vi "PC-PLC.vi"() -> ()   [LabVIEW 2022 SP3]
uses:
  Labview/Globali.vi
panel:
  out "DB20.DBW 254":u16
  out "DB20.DBW 252":u16
  out "DB20.DBW 250":u16
  out "DB20.DBW 248":u16
  out "DB20.DBW 246":u16
  out "DB20.DBW 244":u16
  out "DB20.DBW 242":u16
  out "DB20.DBW 240":u16
  out "DB20.DBW 238":u16
  out "DB20.DBW 236":u16
  out "DB20.DBW 234":u16
  out "DB20.DBW 232":u16
  out "DB20.DBW 230":u16
  out "DB20.DBW 228":u16
  out "DB20.DBW 226":u16
  out "DB20.DBW 224":u16
  out "DB20.DBW 222":u16
  out "DB20.DBW 220":u16
  out "DB20.DBW 218":u16
  out "DB20.DBW 216":u16
  out "DB20.DBW 214":u16
  out "DB20.DBW 212":u16
  out "DB20.DBW 210":u16
  out "DB20.DBW 208":u16
  out "DB20.DBW 206":u16
  out "DB20.DBW 204":u16
  out "DB20.DBW 202":u16
  out "DB20.DBW 200":u16
  out "DB20.DBW 198":u16
  out "DB20.DBW 196":u16
  out "DB20.DBW 194":u16
  out "DB20.DBW 192":u16
  out "DB20.DBW 190":u16
  out "DB20.DBW 188":u16
  out "DB20.DBW 186":u16
  out "DB20.DBW 184":u16
  out "DB20.DBW 182":u16
  out "DB20.DBW 180":u16
  out "DB20.DBW 178":u16
  out "DB20.DBW 176":u16
  out "DB20.DBW 174":u16
  out "DB20.DBW 172":u16
  out "DB20.DBW 170":u16
  out "DB20.DBW 168":u16
  out "DB20.DBW 166":u16
  out "DB20.DBW 164":u16
  out "DB20.DBW 162":u16
  out "DB20.DBW 160":u16
  out "DB20.DBW 158":u16
  out "DB20.DBW 156":u16
  out "DB20.DBW 154":u16
  out "DB20.DBW 152":u16
  out "DB20.DBW 150":u16
  out "DB20.DBW 148":u16
  out "DB20.DBW 146":u16
  out "DB20.DBW 144":u16
  out "DB20.DBW 142":u16
  out "DB20.DBW 140":u16
  out "DB20.DBW 138":u16
  out "DB20.DBW 136":u16
  out "DB20.DBW 134":u16
  out "DB20.DBW 132":u16
  out "DB20.DBW 130":u16
  out "DB20.DBW 128":u16
  out "DB20.DBW 126":u16
  out "DB20.DBW 124":u16
  out "DB20.DBW 122":u16
  out "DB20.DBW 120":u16
  out "DB20.DBW 118":u16
  out "DB20.DBW 116":u16
  out "DB20.DBW 114":u16
  out "DB20.DBW 112":u16
  out "DB20.DBW 110":u16
  out "DB20.DBW 108":u16
  out "DB20.DBW 106":u16
  out "DB20.DBW 104":u16
  out "DB20.DBW 102":u16
  out "DB20.DBW 100":u16
  out "DB20.DBW 98":u16
  out "DB20.DBW 96":u16
  out "DB20.DBW 94":u16
  out "DB20.DBW 92":u16
  out "DB20.DBW 90":u16
  out "DB20.DBW 88":u16
  out "DB20.DBW 86":u16
  out "DB20.DBW 84":u16
  out "DB20.DBW 82":u16
  out "DB20.DBW 80":u16
  out "DB20.DBW 78":u16
  out "DB20.DBW 76":u16
  out "DB20.DBW 74":u16
  out "DB20.DBW 72":u16
  out "DB20.DBW 70":u16
  out "DB20.DBW 68":u16
  out "DB20.DBW 66":u16
  out "DB20.DBW 64":u16
  out "DB20.DBW 62":u16
  out "DB20.DBW 60":u16
  out "DB20.DBW 58":u16
  out "DB20.DBW 56":u16
  out "DB20.DBW 54":u16
  out "DB20.DBW 52":u16
  out "DB20.DBW 50":u16
  out "DB20.DBW 48":u16
  out "DB20.DBW 46":u16
  out "DB20.DBW 44":u16
  out "DB20.DBW 42":u16
  out "DB20.DBW 40":u16
  out "DB20.DBW 38":u16
  out "DB20.DBW 36":u16
  out "DB20.DBW 34":u16
  out "DB20.DBW 32":u16
  out "DB20.DBW 30":u16
  out "DB20.DBW 28":u16
  out "DB20.DBW 26":u16
  out "DB20.DBW 24":u16
  out "DB20.DBW 22":u16
  out "DB20.DBW 20":u16
  out "DB20.DBW 18":u16
  out "DB20.DBW 16":u16
  out "DB20.DBW 14":u16
  out "DB20.DBW 12":u16
  out "DB20.DBW 10":u16
  out "DB20.DBW 8":u16
  out "DB20.DBW 6":u16
  out "DB20.DBW 4":u16
  out "DB20.DBW 2":u16
  out "DB20.DBW 0":u16
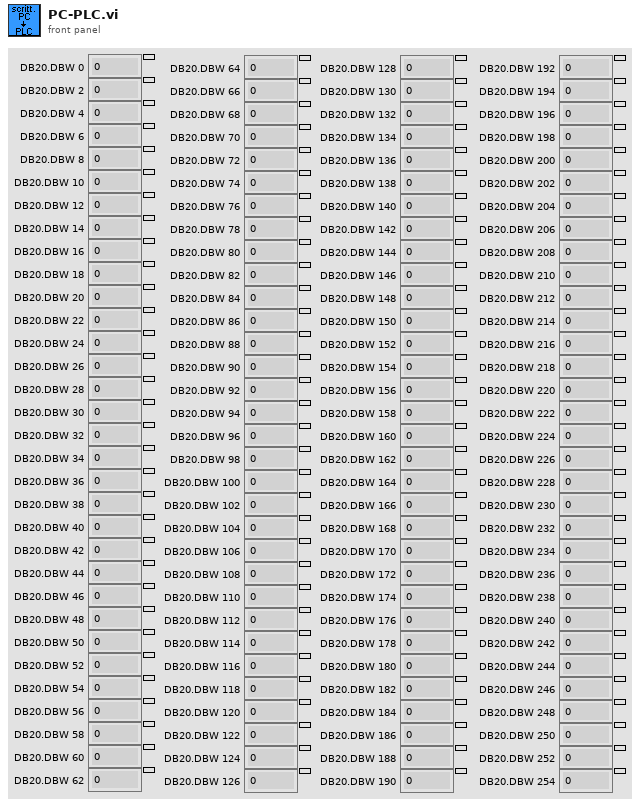
[diagram p1: front panel]
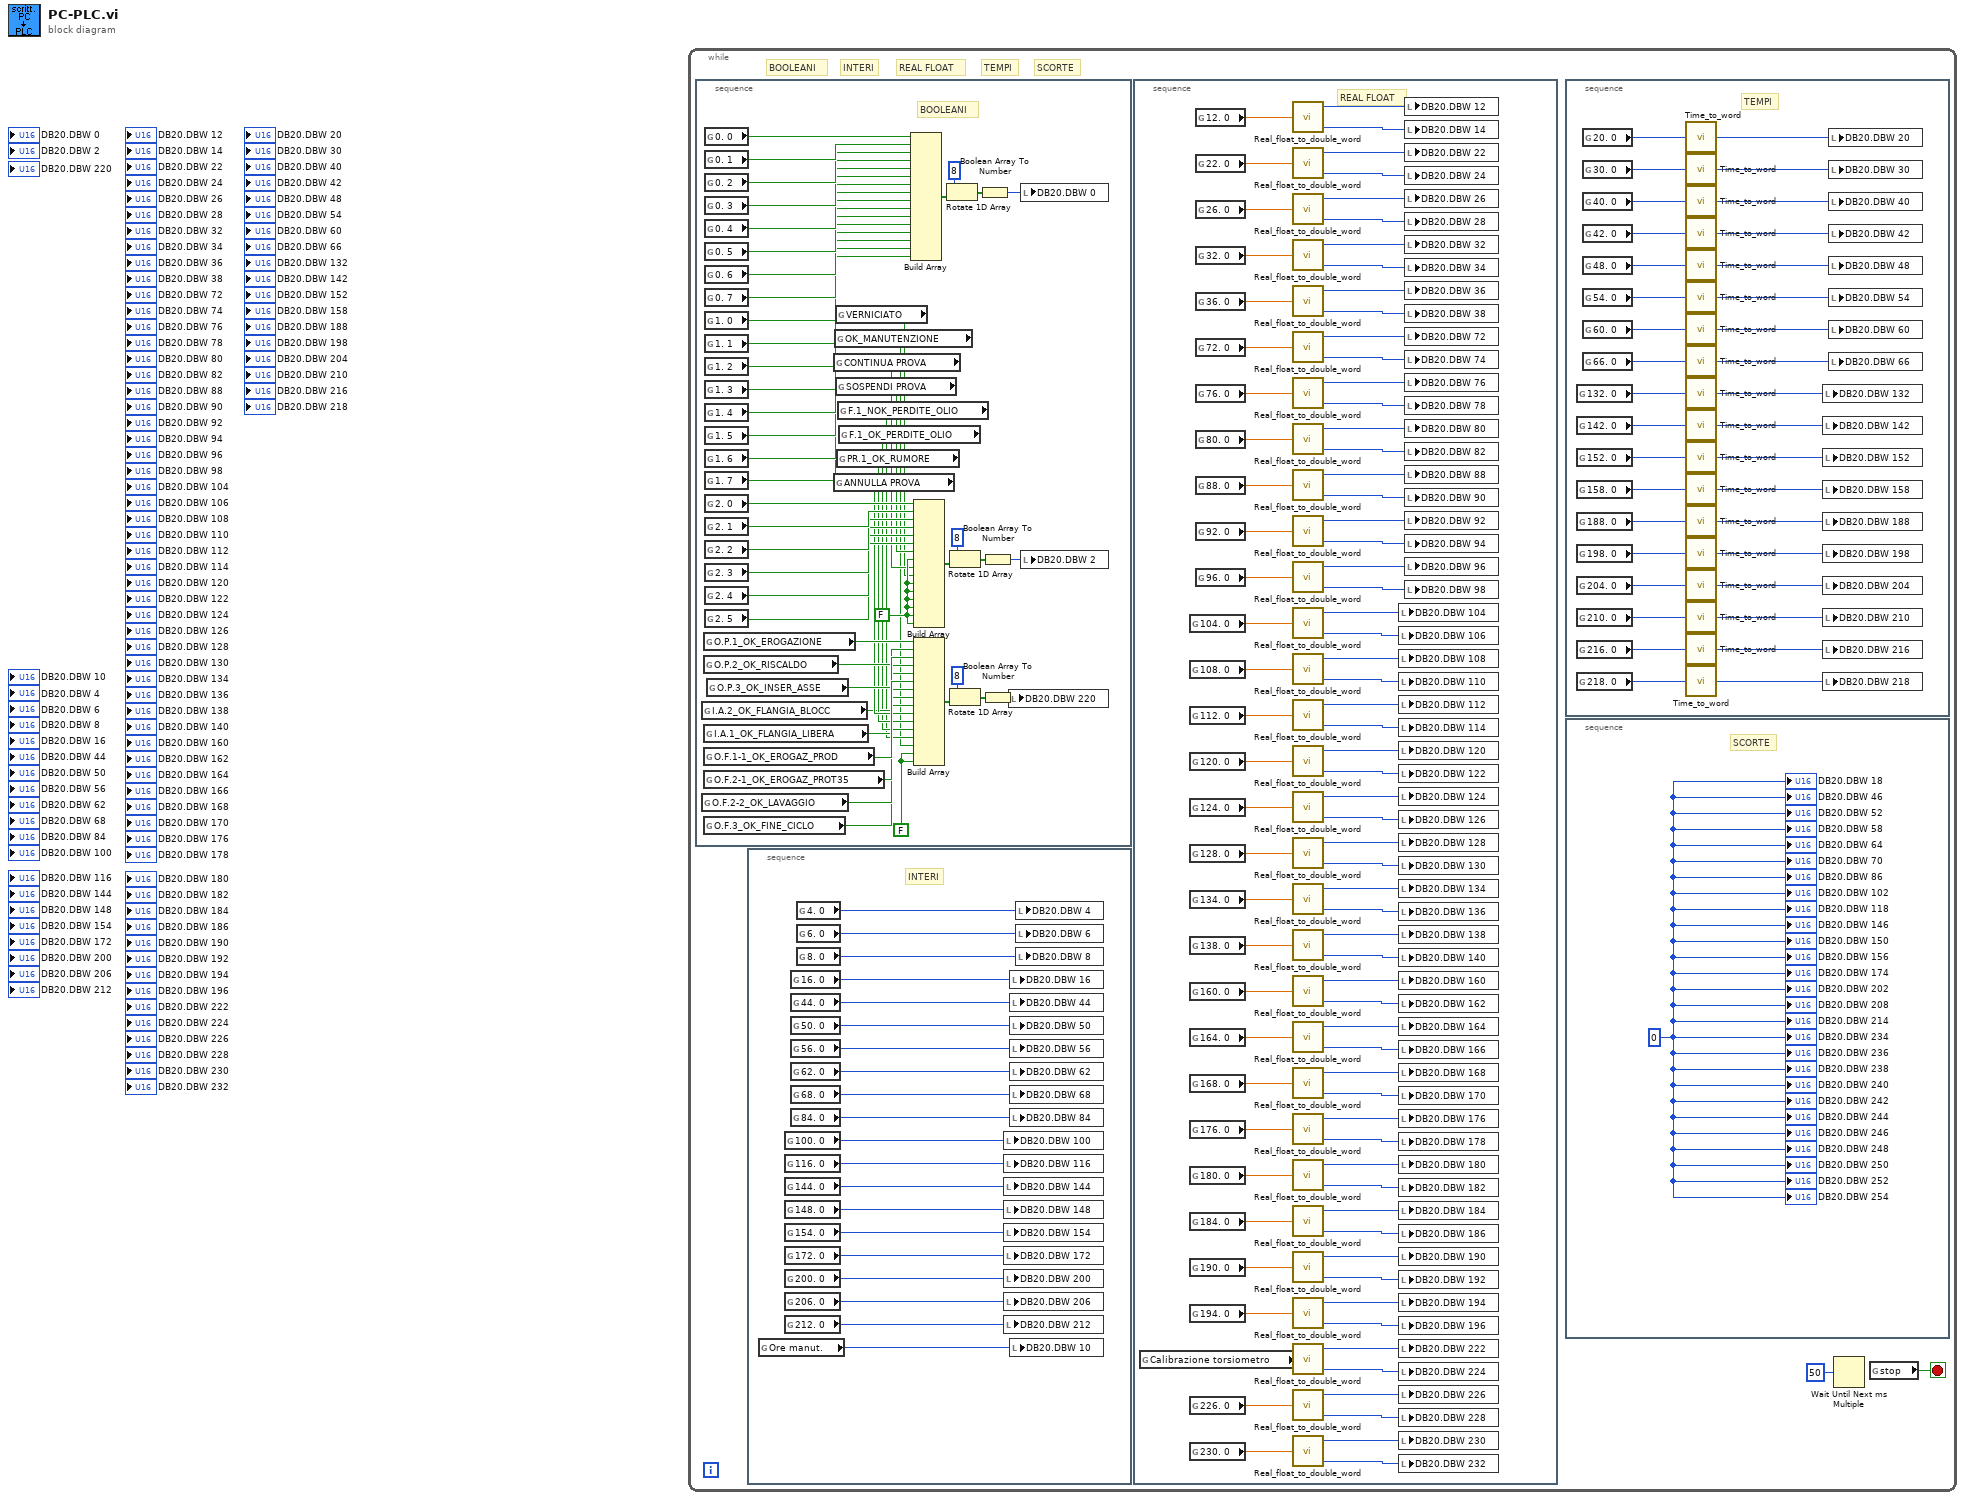
[diagram p0: block diagram]
diagram:
  n1 = while {
    stop <- w1 stop-if-true
    # "SCORTE"
    # "TEMPI"
    # "REAL FLOAT"
    # "INTERI"
    # "BOOLEANI"
    n2 = stacked-sequence {
      frame #0 {
        w6 = FALSE ("element")
        w49 = FALSE ("element")
        # "BOOLEANI"
        n3 = global read "Globali.vi" "I.A.2_OK_FLANGIA_BLOCC"() -> (w11:bool)
        n4 = global read "Globali.vi" "O.F.2-2_OK_LAVAGGIO"() -> (w15:bool)
        n5 = global read "Globali.vi" "O.P.1_OK_EROGAZIONE"() -> (w21:bool)
        n6 = global read "Globali.vi" "O.P.2_OK_RISCALDO"() -> (w22:bool)
        n7 = global read "Globali.vi" "I.A.1_OK_FLANGIA_LIBERA"() -> (w10:bool)
        n8 = global read "Globali.vi" "O.F.1-1_OK_EROGAZ_PROD"() -> (w24:bool)
        n9 = global read "Globali.vi" "O.F.2-1_OK_EROGAZ_PROT35"() -> (w16:bool)
        n10 = global read "Globali.vi" "O.F.3_OK_FINE_CICLO"() -> (w14:bool)
        n11 = global read "Globali.vi" "0. 0"() -> (w48:bool)
        n12 = global read "Globali.vi" "0. 1"() -> (w47:bool)
        n13 = global read "Globali.vi" "0. 2"() -> (w46:bool)
        n14 = global read "Globali.vi" "0. 3"() -> (w45:bool)
        n15 = global read "Globali.vi" "0. 4"() -> (w44:bool)
        n16 = global read "Globali.vi" "0. 5"() -> (w43:bool)
        n17 = global read "Globali.vi" "0. 6"() -> (w42:bool)
        n18 = global read "Globali.vi" "0. 7"() -> (w41:bool)
        n19 = global read "Globali.vi" "1. 0"() -> (w40:bool)
        n20 = global read "Globali.vi" "1. 1"() -> (w39:bool)
        n21 = global read "Globali.vi" "1. 2"() -> (w38:bool)
        n22 = global read "Globali.vi" "1. 3"() -> (w37:bool)
        n23 = global read "Globali.vi" "1. 4"() -> (w36:bool)
        n24 = global read "Globali.vi" "1. 5"() -> (w35:bool)
        n25 = global read "Globali.vi" "1. 6"() -> (w34:bool)
        n26 = global read "Globali.vi" "1. 7"() -> (w33:bool)
        n27 = global read "Globali.vi" "2. 0"() -> (w32:bool)
        n28 = global read "Globali.vi" "2. 1"() -> (w31:bool)
        n29 = global read "Globali.vi" "2. 2"() -> (w30:bool)
        n30 = global read "Globali.vi" "2. 3"() -> (w29:bool)
        n31 = global read "Globali.vi" "2. 4"() -> (w28:bool)
        n32 = global read "Globali.vi" "2. 5"() -> (w27:bool)
        n33 = global read "Globali.vi" "O.P.3_OK_INSER_ASSE"() -> (w23:bool)
        n34 = global read "Globali.vi" "CONTINUA PROVA"() -> (w5:bool)
        n35 = global read "Globali.vi" "ANNULLA PROVA"() -> (w13:bool)
        n36 = global read "Globali.vi" "OK_MANUTENZIONE"() -> (w4:bool)
        n37 = global read "Globali.vi" "VERNICIATO"() -> (w3:bool)
        n38 = global read "Globali.vi" "SOSPENDI PROVA"() -> (w7:bool)
        n39 = global read "Globali.vi" "PR.1_OK_RUMORE"() -> (w12:bool)
        n40 = global read "Globali.vi" "F.1_NOK_PERDITE_OLIO"() -> (w8:bool)
        n41 = global read "Globali.vi" "F.1_OK_PERDITE_OLIO"() -> (w9:bool)
        n42 = Build Array(w48, w47, w46, w45, w44, w43, w42, w41, w40, w39, w38, w37, w36, w35, w34, w33) -> (w51:bool[])
        n43 = Build Array(w32, w31, w30, w29, w28, w27, w7, w49, w5, w3, w49, w49, w49, w49, w49, w49) -> (w53:bool[])
        n44 = Build Array(w21, w22, w23, w11, w10, w24, w16, w15, w14, w13, w12, w9, w8, w4, w6, w6) -> (w19:bool[])
        n45 = Rotate 1D Array(1:w51, 2:8 ("n")) -> (0:w54:bool[])
        n46 = Rotate 1D Array(1:w53, 2:8 ("n")) -> (0:w55:bool[])
        n47 = Rotate 1D Array(1:w19, 2:8 ("n")) -> (0:w18:bool[])
        n48 = Boolean Array To Number(Boolean array=w54) -> (number=w26:u32)
        n49 = Boolean Array To Number(Boolean array=w55) -> (number=w25:u32)
        n50 = Boolean Array To Number(Boolean array=w18) -> (number=w17:u32)
        n51 = local write "DB20.DBW 220"(w17) -> ()
        n52 = local write "DB20.DBW 0"(w26) -> ()
        n53 = local write "DB20.DBW 2"(w25) -> ()
      }
    }
    n54 = stacked-sequence {
      frame #0 {
        # "INTERI"
        n55 = global read "Globali.vi" "Ore manut."() -> (w93:i16)
        n56 = global read "Globali.vi" "100. 0"() -> (w102:i16)
        n57 = global read "Globali.vi" "116. 0"() -> (w101:i16)
        n58 = global read "Globali.vi" "144. 0"() -> (w100:i16)
        n59 = global read "Globali.vi" "148. 0"() -> (w99:i16)
        n60 = global read "Globali.vi" "154. 0"() -> (w98:i16)
        n61 = global read "Globali.vi" "172. 0"() -> (w97:i16)
        n62 = global read "Globali.vi" "200. 0"() -> (w96:i16)
        n63 = global read "Globali.vi" "206. 0"() -> (w95:i16)
        n64 = global read "Globali.vi" "212. 0"() -> (w94:i16)
        n65 = global read "Globali.vi" "16. 0"() -> (w109:i16)
        n66 = global read "Globali.vi" "44. 0"() -> (w108:i16)
        n67 = global read "Globali.vi" "50. 0"() -> (w107:i16)
        n68 = global read "Globali.vi" "56. 0"() -> (w106:i16)
        n69 = global read "Globali.vi" "62. 0"() -> (w105:i16)
        n70 = global read "Globali.vi" "68. 0"() -> (w104:i16)
        n71 = global read "Globali.vi" "84. 0"() -> (w103:i16)
        n72 = global read "Globali.vi" "4. 0"() -> (w112:i16)
        n73 = global read "Globali.vi" "6. 0"() -> (w111:i16)
        n74 = global read "Globali.vi" "8. 0"() -> (w110:i16)
        n75 = local write "DB20.DBW 100"(w102) -> ()
        n76 = local write "DB20.DBW 116"(w101) -> ()
        n77 = local write "DB20.DBW 144"(w100) -> ()
        n78 = local write "DB20.DBW 148"(w99) -> ()
        n79 = local write "DB20.DBW 154"(w98) -> ()
        n80 = local write "DB20.DBW 172"(w97) -> ()
        n81 = local write "DB20.DBW 200"(w96) -> ()
        n82 = local write "DB20.DBW 206"(w95) -> ()
        n83 = local write "DB20.DBW 212"(w94) -> ()
        n84 = local write "DB20.DBW 16"(w109) -> ()
        n85 = local write "DB20.DBW 44"(w108) -> ()
        n86 = local write "DB20.DBW 50"(w107) -> ()
        n87 = local write "DB20.DBW 56"(w106) -> ()
        n88 = local write "DB20.DBW 62"(w105) -> ()
        n89 = local write "DB20.DBW 68"(w104) -> ()
        n90 = local write "DB20.DBW 84"(w103) -> ()
        n91 = local write "DB20.DBW 10"(w93) -> ()
        n92 = local write "DB20.DBW 4"(w112) -> ()
        n93 = local write "DB20.DBW 6"(w111) -> ()
        n94 = local write "DB20.DBW 8"(w110) -> ()
      }
    }
    n95 = stacked-sequence {
      frame #0 {
        # "REAL FLOAT"
        n96 = global read "Globali.vi" "Calibrazione torsiometro"() -> (w119:sgl)
        n97 = global read "Globali.vi" "104. 0"() -> (w191:sgl)
        n98 = global read "Globali.vi" "108. 0"() -> (w190:sgl)
        n99 = global read "Globali.vi" "112. 0"() -> (w176:sgl)
        n100 = global read "Globali.vi" "120. 0"() -> (w177:sgl)
        n101 = global read "Globali.vi" "124. 0"() -> (w178:sgl)
        n102 = global read "Globali.vi" "128. 0"() -> (w179:sgl)
        n103 = global read "Globali.vi" "134. 0"() -> (w180:sgl)
        n104 = global read "Globali.vi" "138. 0"() -> (w181:sgl)
        n105 = global read "Globali.vi" "160. 0"() -> (w182:sgl)
        n106 = global read "Globali.vi" "164. 0"() -> (w183:sgl)
        n107 = global read "Globali.vi" "168. 0"() -> (w184:sgl)
        n108 = global read "Globali.vi" "176. 0"() -> (w185:sgl)
        n109 = global read "Globali.vi" "180. 0"() -> (w186:sgl)
        n110 = global read "Globali.vi" "184. 0"() -> (w187:sgl)
        n111 = global read "Globali.vi" "190. 0"() -> (w188:sgl)
        n112 = global read "Globali.vi" "194. 0"() -> (w189:sgl)
        n113 = global read "Globali.vi" "226. 0"() -> (w113:sgl)
        n114 = global read "Globali.vi" "230. 0"() -> (w118:sgl)
        n115 = global read "Globali.vi" "12. 0"() -> (w202:sgl)
        n116 = global read "Globali.vi" "22. 0"() -> (w201:sgl)
        n117 = global read "Globali.vi" "26. 0"() -> (w200:sgl)
        n118 = global read "Globali.vi" "32. 0"() -> (w199:sgl)
        n119 = global read "Globali.vi" "36. 0"() -> (w198:sgl)
        n120 = global read "Globali.vi" "72. 0"() -> (w197:sgl)
        n121 = global read "Globali.vi" "76. 0"() -> (w196:sgl)
        n122 = global read "Globali.vi" "80. 0"() -> (w195:sgl)
        n123 = global read "Globali.vi" "88. 0"() -> (w194:sgl)
        n124 = global read "Globali.vi" "92. 0"() -> (w193:sgl)
        n125 = global read "Globali.vi" "96. 0"() -> (w192:sgl)
        n126 = call "Real_float_to_double_word.vi"("Real float"=w202) -> ("Seconda word"=w174:u16, "Prima word"=w175:u16)  [unwired: 3 in]
        n127 = call "Real_float_to_double_word.vi"("Real float"=w201) -> ("Seconda word"=w172:u16, "Prima word"=w173:u16)  [unwired: 3 in]
        n128 = call "Real_float_to_double_word.vi"("Real float"=w200) -> ("Seconda word"=w160:u16, "Prima word"=w161:u16)  [unwired: 3 in]
        n129 = call "Real_float_to_double_word.vi"("Real float"=w199) -> ("Seconda word"=w158:u16, "Prima word"=w159:u16)  [unwired: 3 in]
        n130 = call "Real_float_to_double_word.vi"("Real float"=w198) -> ("Seconda word"=w156:u16, "Prima word"=w157:u16)  [unwired: 3 in]
        n131 = call "Real_float_to_double_word.vi"("Real float"=w197) -> ("Seconda word"=w154:u16, "Prima word"=w155:u16)  [unwired: 3 in]
        n132 = call "Real_float_to_double_word.vi"("Real float"=w196) -> ("Seconda word"=w146:u16, "Prima word"=w147:u16)  [unwired: 3 in]
        n133 = call "Real_float_to_double_word.vi"("Real float"=w195) -> ("Seconda word"=w144:u16, "Prima word"=w145:u16)  [unwired: 3 in]
        n134 = call "Real_float_to_double_word.vi"("Real float"=w194) -> ("Seconda word"=w142:u16, "Prima word"=w143:u16)  [unwired: 3 in]
        n135 = call "Real_float_to_double_word.vi"("Real float"=w193) -> ("Seconda word"=w140:u16, "Prima word"=w141:u16)  [unwired: 3 in]
        n136 = call "Real_float_to_double_word.vi"("Real float"=w192) -> ("Seconda word"=w138:u16, "Prima word"=w139:u16)  [unwired: 3 in]
        n137 = call "Real_float_to_double_word.vi"("Real float"=w191) -> ("Seconda word"=w136:u16, "Prima word"=w137:u16)  [unwired: 3 in]
        n138 = call "Real_float_to_double_word.vi"("Real float"=w190) -> ("Seconda word"=w134:u16, "Prima word"=w135:u16)  [unwired: 3 in]
        n139 = call "Real_float_to_double_word.vi"("Real float"=w176) -> ("Seconda word"=w122:u16, "Prima word"=w133:u16)  [unwired: 3 in]
        n140 = call "Real_float_to_double_word.vi"("Real float"=w177) -> ("Seconda word"=w124:u16, "Prima word"=w123:u16)  [unwired: 3 in]
        n141 = call "Real_float_to_double_word.vi"("Real float"=w178) -> ("Seconda word"=w126:u16, "Prima word"=w125:u16)  [unwired: 3 in]
        n142 = call "Real_float_to_double_word.vi"("Real float"=w179) -> ("Seconda word"=w128:u16, "Prima word"=w127:u16)  [unwired: 3 in]
        n143 = call "Real_float_to_double_word.vi"("Real float"=w180) -> ("Seconda word"=w130:u16, "Prima word"=w129:u16)  [unwired: 3 in]
        n144 = call "Real_float_to_double_word.vi"("Real float"=w181) -> ("Seconda word"=w132:u16, "Prima word"=w131:u16)  [unwired: 3 in]
        n145 = call "Real_float_to_double_word.vi"("Real float"=w182) -> ("Seconda word"=w149:u16, "Prima word"=w148:u16)  [unwired: 3 in]
        n146 = call "Real_float_to_double_word.vi"("Real float"=w183) -> ("Seconda word"=w151:u16, "Prima word"=w150:u16)  [unwired: 3 in]
        n147 = call "Real_float_to_double_word.vi"("Real float"=w184) -> ("Seconda word"=w153:u16, "Prima word"=w152:u16)  [unwired: 3 in]
        n148 = call "Real_float_to_double_word.vi"("Real float"=w185) -> ("Seconda word"=w163:u16, "Prima word"=w162:u16)  [unwired: 3 in]
        n149 = call "Real_float_to_double_word.vi"("Real float"=w186) -> ("Seconda word"=w165:u16, "Prima word"=w164:u16)  [unwired: 3 in]
        n150 = call "Real_float_to_double_word.vi"("Real float"=w187) -> ("Seconda word"=w167:u16, "Prima word"=w166:u16)  [unwired: 3 in]
        n151 = call "Real_float_to_double_word.vi"("Real float"=w188) -> ("Seconda word"=w169:u16, "Prima word"=w168:u16)  [unwired: 3 in]
        n152 = call "Real_float_to_double_word.vi"("Real float"=w189) -> ("Seconda word"=w170:u16, "Prima word"=w171:u16)  [unwired: 3 in]
        n153 = call "Real_float_to_double_word.vi"("Real float"=w119) -> ("Seconda word"=w120:u16, "Prima word"=w121:u16)  [unwired: 3 in]
        n154 = call "Real_float_to_double_word.vi"("Real float"=w113) -> ("Seconda word"=w115:u16, "Prima word"=w114:u16)  [unwired: 3 in]
        n155 = call "Real_float_to_double_word.vi"("Real float"=w118) -> ("Seconda word"=w117:u16, "Prima word"=w116:u16)  [unwired: 3 in]
        n156 = local write "DB20.DBW 104"(w137) -> ()
        n157 = local write "DB20.DBW 106"(w136) -> ()
        n158 = local write "DB20.DBW 108"(w135) -> ()
        n159 = local write "DB20.DBW 110"(w134) -> ()
        n160 = local write "DB20.DBW 112"(w133) -> ()
        n161 = local write "DB20.DBW 114"(w122) -> ()
        n162 = local write "DB20.DBW 120"(w123) -> ()
        n163 = local write "DB20.DBW 122"(w124) -> ()
        n164 = local write "DB20.DBW 124"(w125) -> ()
        n165 = local write "DB20.DBW 126"(w126) -> ()
        n166 = local write "DB20.DBW 128"(w127) -> ()
        n167 = local write "DB20.DBW 130"(w128) -> ()
        n168 = local write "DB20.DBW 134"(w129) -> ()
        n169 = local write "DB20.DBW 136"(w130) -> ()
        n170 = local write "DB20.DBW 138"(w131) -> ()
        n171 = local write "DB20.DBW 140"(w132) -> ()
        n172 = local write "DB20.DBW 160"(w148) -> ()
        n173 = local write "DB20.DBW 162"(w149) -> ()
        n174 = local write "DB20.DBW 164"(w150) -> ()
        n175 = local write "DB20.DBW 166"(w151) -> ()
        n176 = local write "DB20.DBW 168"(w152) -> ()
        n177 = local write "DB20.DBW 170"(w153) -> ()
        n178 = local write "DB20.DBW 176"(w162) -> ()
        n179 = local write "DB20.DBW 178"(w163) -> ()
        n180 = local write "DB20.DBW 180"(w164) -> ()
        n181 = local write "DB20.DBW 182"(w165) -> ()
        n182 = local write "DB20.DBW 184"(w166) -> ()
        n183 = local write "DB20.DBW 186"(w167) -> ()
        n184 = local write "DB20.DBW 190"(w168) -> ()
        n185 = local write "DB20.DBW 192"(w169) -> ()
        n186 = local write "DB20.DBW 194"(w171) -> ()
        n187 = local write "DB20.DBW 196"(w170) -> ()
        n188 = local write "DB20.DBW 222"(w121) -> ()
        n189 = local write "DB20.DBW 224"(w120) -> ()
        n190 = local write "DB20.DBW 226"(w114) -> ()
        n191 = local write "DB20.DBW 228"(w115) -> ()
        n192 = local write "DB20.DBW 230"(w116) -> ()
        n193 = local write "DB20.DBW 232"(w117) -> ()
        n194 = local write "DB20.DBW 12"(w175) -> ()
        n195 = local write "DB20.DBW 14"(w174) -> ()
        n196 = local write "DB20.DBW 22"(w173) -> ()
        n197 = local write "DB20.DBW 24"(w172) -> ()
        n198 = local write "DB20.DBW 26"(w161) -> ()
        n199 = local write "DB20.DBW 28"(w160) -> ()
        n200 = local write "DB20.DBW 32"(w159) -> ()
        n201 = local write "DB20.DBW 34"(w158) -> ()
        n202 = local write "DB20.DBW 36"(w157) -> ()
        n203 = local write "DB20.DBW 38"(w156) -> ()
        n204 = local write "DB20.DBW 72"(w155) -> ()
        n205 = local write "DB20.DBW 74"(w154) -> ()
        n206 = local write "DB20.DBW 76"(w147) -> ()
        n207 = local write "DB20.DBW 78"(w146) -> ()
        n208 = local write "DB20.DBW 80"(w145) -> ()
        n209 = local write "DB20.DBW 82"(w144) -> ()
        n210 = local write "DB20.DBW 88"(w143) -> ()
        n211 = local write "DB20.DBW 90"(w142) -> ()
        n212 = local write "DB20.DBW 92"(w141) -> ()
        n213 = local write "DB20.DBW 94"(w140) -> ()
        n214 = local write "DB20.DBW 96"(w139) -> ()
        n215 = local write "DB20.DBW 98"(w138) -> ()
      }
    }
    n216 = stacked-sequence {
      frame #0 {
        # "TEMPI"
        n217 = global read "Globali.vi" "132. 0"() -> (w83:u16)
        n218 = global read "Globali.vi" "142. 0"() -> (w82:u16)
        n219 = global read "Globali.vi" "152. 0"() -> (w81:u16)
        n220 = global read "Globali.vi" "158. 0"() -> (w80:u16)
        n221 = global read "Globali.vi" "188. 0"() -> (w79:u16)
        n222 = global read "Globali.vi" "198. 0"() -> (w78:u16)
        n223 = global read "Globali.vi" "204. 0"() -> (w77:u16)
        n224 = global read "Globali.vi" "210. 0"() -> (w76:u16)
        n225 = global read "Globali.vi" "216. 0"() -> (w75:u16)
        n226 = global read "Globali.vi" "218. 0"() -> (w74:u16)
        n227 = global read "Globali.vi" "20. 0"() -> (w91:u16)
        n228 = global read "Globali.vi" "30. 0"() -> (w90:u16)
        n229 = global read "Globali.vi" "40. 0"() -> (w89:u16)
        n230 = global read "Globali.vi" "42. 0"() -> (w88:u16)
        n231 = global read "Globali.vi" "48. 0"() -> (w87:u16)
        n232 = global read "Globali.vi" "54. 0"() -> (w86:u16)
        n233 = global read "Globali.vi" "60. 0"() -> (w85:u16)
        n234 = global read "Globali.vi" "66. 0"() -> (w84:u16)
        n235 = call "Time_to_word.vi"("Tempo (sec)"=w91) -> ("word"=w73:u16)  [unwired: 4 in]
        n236 = call "Time_to_word.vi"("Tempo (sec)"=w90) -> ("word"=w71:u16)  [unwired: 4 in]
        n237 = call "Time_to_word.vi"("Tempo (sec)"=w89) -> ("word"=w70:u16)  [unwired: 4 in]
        n238 = call "Time_to_word.vi"("Tempo (sec)"=w88) -> ("word"=w69:u16)  [unwired: 4 in]
        n239 = call "Time_to_word.vi"("Tempo (sec)"=w87) -> ("word"=w68:u16)  [unwired: 4 in]
        n240 = call "Time_to_word.vi"("Tempo (sec)"=w86) -> ("word"=w67:u16)  [unwired: 4 in]
        n241 = call "Time_to_word.vi"("Tempo (sec)"=w85) -> ("word"=w66:u16)  [unwired: 4 in]
        n242 = call "Time_to_word.vi"("Tempo (sec)"=w84) -> ("word"=w65:u16)  [unwired: 4 in]
        n243 = call "Time_to_word.vi"("Tempo (sec)"=w83) -> ("word"=w64:u16)  [unwired: 4 in]
        n244 = call "Time_to_word.vi"("Tempo (sec)"=w82) -> ("word"=w63:u16)  [unwired: 4 in]
        n245 = call "Time_to_word.vi"("Tempo (sec)"=w81) -> ("word"=w62:u16)  [unwired: 4 in]
        n246 = call "Time_to_word.vi"("Tempo (sec)"=w80) -> ("word"=w61:u16)  [unwired: 4 in]
        n247 = call "Time_to_word.vi"("Tempo (sec)"=w79) -> ("word"=w60:u16)  [unwired: 4 in]
        n248 = call "Time_to_word.vi"("Tempo (sec)"=w78) -> ("word"=w59:u16)  [unwired: 4 in]
        n249 = call "Time_to_word.vi"("Tempo (sec)"=w77) -> ("word"=w58:u16)  [unwired: 4 in]
        n250 = call "Time_to_word.vi"("Tempo (sec)"=w76) -> ("word"=w57:u16)  [unwired: 4 in]
        n251 = call "Time_to_word.vi"("Tempo (sec)"=w75) -> ("word"=w56:u16)  [unwired: 4 in]
        n252 = call "Time_to_word.vi"("Tempo (sec)"=w74) -> ("word"=w72:u16)  [unwired: 4 in]
        n253 = local write "DB20.DBW 132"(w64) -> ()
        n254 = local write "DB20.DBW 142"(w63) -> ()
        n255 = local write "DB20.DBW 152"(w62) -> ()
        n256 = local write "DB20.DBW 158"(w61) -> ()
        n257 = local write "DB20.DBW 188"(w60) -> ()
        n258 = local write "DB20.DBW 198"(w59) -> ()
        n259 = local write "DB20.DBW 204"(w58) -> ()
        n260 = local write "DB20.DBW 210"(w57) -> ()
        n261 = local write "DB20.DBW 216"(w56) -> ()
        n262 = local write "DB20.DBW 218"(w72) -> ()
        n263 = local write "DB20.DBW 20"(w73) -> ()
        n264 = local write "DB20.DBW 30"(w71) -> ()
        n265 = local write "DB20.DBW 40"(w70) -> ()
        n266 = local write "DB20.DBW 42"(w69) -> ()
        n267 = local write "DB20.DBW 48"(w68) -> ()
        n268 = local write "DB20.DBW 54"(w67) -> ()
        n269 = local write "DB20.DBW 60"(w66) -> ()
        n270 = local write "DB20.DBW 66"(w65) -> ()
      }
    }
    n271 = stacked-sequence {
      frame #0 {
        w92 = u16 0 ("DB20.DBW 220")
        # "SCORTE"
        "DB20.DBW 234" <- w92
        "DB20.DBW 236" <- w92
        "DB20.DBW 238" <- w92
        "DB20.DBW 240" <- w92
        "DB20.DBW 242" <- w92
        "DB20.DBW 244" <- w92
        "DB20.DBW 246" <- w92
        "DB20.DBW 248" <- w92
        "DB20.DBW 250" <- w92
        "DB20.DBW 252" <- w92
        "DB20.DBW 254" <- w92
        "DB20.DBW 18" <- w92
        "DB20.DBW 46" <- w92
        "DB20.DBW 52" <- w92
        "DB20.DBW 64" <- w92
        "DB20.DBW 70" <- w92
        "DB20.DBW 86" <- w92
        "DB20.DBW 102" <- w92
        "DB20.DBW 118" <- w92
        "DB20.DBW 146" <- w92
        "DB20.DBW 156" <- w92
        "DB20.DBW 174" <- w92
        "DB20.DBW 202" <- w92
        "DB20.DBW 208" <- w92
        "DB20.DBW 214" <- w92
        "DB20.DBW 150" <- w92
        "DB20.DBW 58" <- w92
      }
    }
    n272 = Wait Until Next ms Multiple(millisecond multiple=u32 50) -> ()  [unwired: 1 out]
    n273 = global read "Globali.vi" "stop"() -> (w1:bool)
  }
